vi "多布尔输入条件结构.vi"() -> ()   [LabVIEW 2022 SP3]
doc: "本VI是为《我和LabVIEW》一书编写的示例。\n关于本书的介绍请参考网页：\nhttp://ruanqizhen.spaces.live.com/blog/cns!5852D4F797C53FB6!4310.entry"
panel:
  out "数字":u32
  in  "b":bool
  in  "a":bool
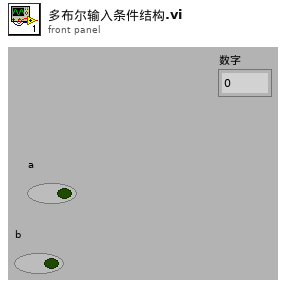
[diagram p1: front panel]
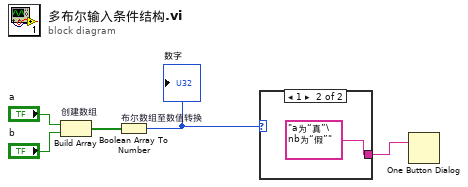
[diagram p0: block diagram]
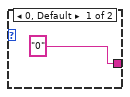
[diagram p2: hidden frame]
diagram:
  n1 = Build Array "创建数组"("a", "b") -> (w3:bool[])
  n2 = Boolean Array To Number "布尔数组至数值转换"(Boolean array=w3) -> (number=w2:u32)
  "数字" <- w2
  n3 = case shown="1" w2 {
    tunnel: ["0" "a为“真”\nb为“假”"] -> w1
    frame 0, Default {
    }
    frame 1 {
    }
  }
  n4 = One Button Dialog(message=w1) -> ()  [unwired: 1 in, 1 out]
